vi "Teleop.vi"(10 "Match Info":T2={"Autonomous Elapsed Seconds"=0.0, "TeleOp Elapsed Seconds"=300.781, "Disabled Elapsed Seconds"=0.999, "Visited Autonomous"=FALSE, "Visited TeleOp"=TRUE, "Visited Disabled"=TRUE, "Autonomous Settings"={"Autonomous Style"=enum."Independent", "VI Refnum"=refnum}}, 11 "Call Context":T3=enum."Execute") -> ()   [LabVIEW 2016]
doc: "This VI is called for each TeleOp packet received from the DS where the robot is not disabled. It is often used to read from the joysticks and update I/O or to update setpoints for timed control loops. It should complete and return within 20 milliseconds or it may miss DS packets."
uses:
  <vilib>/Rock Robotics/WPI/DriverStation/WPI_DriverStationDerivedRobotMode.ctl
  <vilib>/Rock Robotics/WPI/DriverStation/WPI_DriverStationMatch Info.ctl
  <vilib>/Rock Robotics/WPI/Solenoid/WPI_SolenoidValue.ctl
  <vilib>/Rock Robotics/WPI/Utilities/WPI_GetSetVariantRefNum.vi
  <vilib>/Rock Robotics/Network Tables/NT Write Boolean Array.vi
  <vilib>/Rock Robotics/Network Tables/NT Write Numeric Array.vi
  <vilib>/Rock Robotics/Network Tables/NT Read Boolean.vi
  <vilib>/Rock Robotics/Network Tables/NT Read Number.vi
  <vilib>/Rock Robotics/Network Tables/NT Read String.vi
  <vilib>/Rock Robotics/WPI/Solenoid/WPI_SolenoidSetEnum.vi
  <vilib>/addons/control/pid/pid.llb/PID (DBL).vi
  <vilib>/addons/control/pid/NI_PID_pid.lvlib
panel:
  in  "PID gains":T1={"proportional gain (Kc)"=2.0, "integral time (Ti, min)"=0.02, "derivative time (Td, min)"=0.0}
  out "Output":dbl(graph)=-6.138070230177018
  out "Process Variable":dbl(graph)=160.15643445714286
  out "Setpoint":dbl(graph)=162.0
  in  "setpoint":dbl(slide)=162.0 scale=0.0..270.0
  in  "Solenoid Timer":dbl=1.0 caption="Time Target (s)"
  out "Solenoid Voltage":dbl=24.5625
  out "Input Voltage":dbl=11.45
  out "Power":dbl
  out "current (A)":dbl
  out "Degrees":dbl=160.15643445714286
  out "Voltage":dbl=2.808837603
  out "Sample Slider 0":dbl(slide) scale=0.0..5.0
  out "Sample Boolean 1":bool
  out "Sample Boolean 0":bool
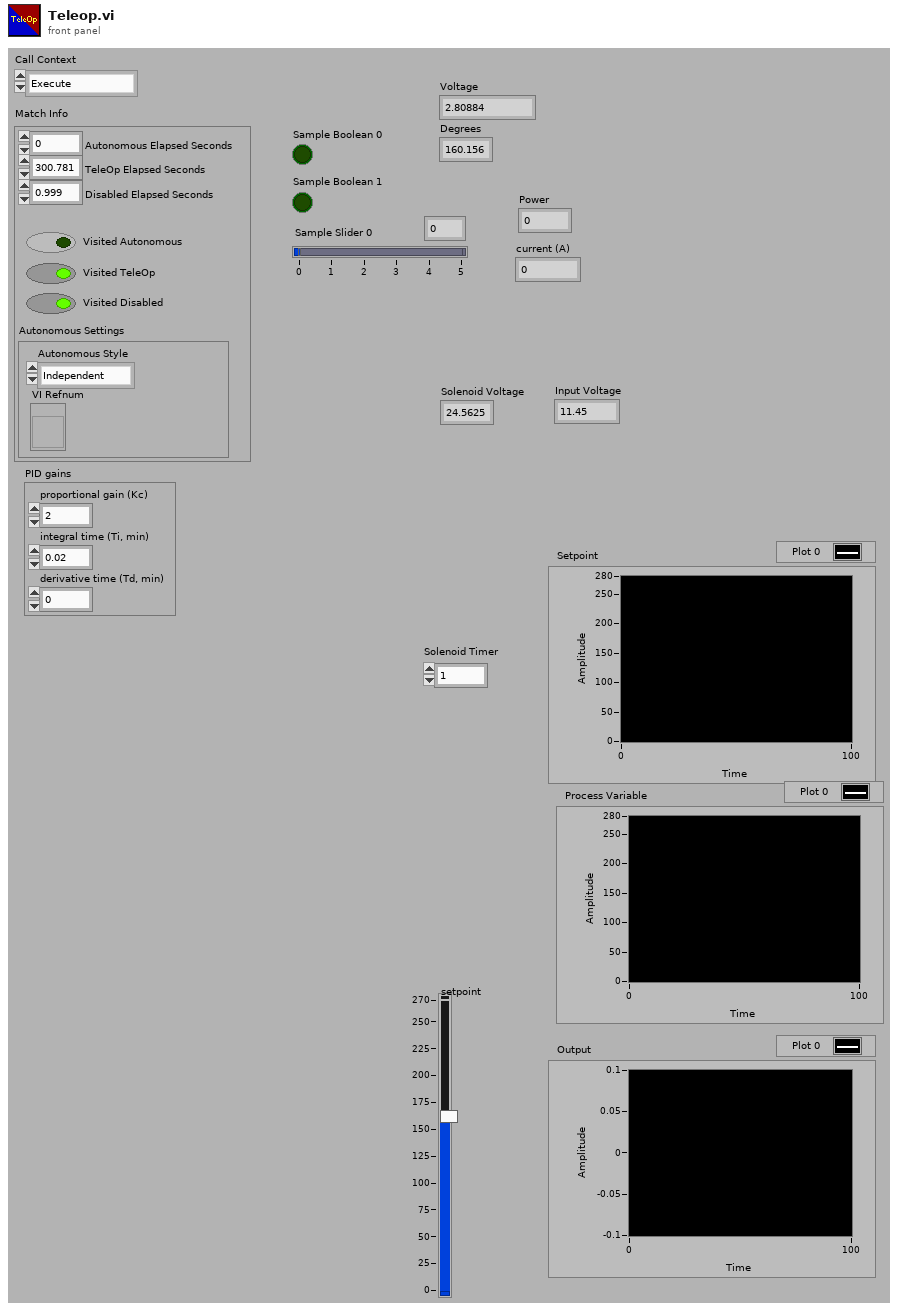
[diagram p1: front panel]
types:
  T1 = cluster{"proportional gain (Kc)":dbl, "integral time (Ti, min)":dbl, "derivative time (Td, min)":dbl}
  T2 = typedef "WPI_DriverStationMatch Info.ctl" = cluster{"Autonomous Elapsed Seconds":dbl, "TeleOp Elapsed Seconds":dbl, "Disabled Elapsed Seconds":dbl, "Visited Autonomous":bool, "Visited TeleOp":bool, "Visited Disabled":bool, "Autonomous Settings":cluster{"Autonomous Style":enum16{"Iterative", "Independent"}, "VI Refnum":refnum<vi>}}
  T3 = typedef "WPI_DriverStationDerivedRobotMode.ctl" = enum16{"Init", "Execute", "Stop"}
  T4 = typedef "WPI_SolenoidValue.ctl" = enum16{"Off", "On", "Forward", "Reverse"}
  T5 = typedef "WPI_RobotDriveDevRef.ctl" = cluster{"DevStatus":errorcluster, "Motors[]":T6[], "Square Inputs":bool, "Max Output":dbl}
  T6 = typedef "WPI_MotorControlDeviceRef.ctl" = cluster{"DeviceStatus":errorcluster, "Type":T7, "PWM":cluster{"PWM Channel":T8, "DeadBand":T9}, "CAN":cluster{"Device Number":u8, "SetOutput VI Ref":variant, "GetOutput VI Ref":variant, "Enable VI Ref":variant, "Disable VI Ref":variant, "Data":variant}, "Invert":bool}
  T7 = typedef "WPI_MotorControlType.ctl" = enum16{"PWM", "CAN"}
  T8 = typedef "FPGA_DIOPWMChannel.ctl" = enum8{"PWM 0", "PWM 1", "PWM 2", "PWM 3", "PWM 4", "PWM 5", "PWM 6", "PWM 7", "PWM 8", "PWM 9", "PWM MXP 0", "PWM MXP 1", "PWM MXP 2", "PWM MXP 3", "PWM MXP 4", "PWM MXP 5", "PWM MXP 6", "PWM MXP 7", "PWM MXP 8", "PWM MXP 9", "Invalid"}
  T9 = typedef "WPI_PWMDeadband.ctl" = cluster{"Name":string, "maxPositivePwm":i32, "minPositivePwm":i32, "centerPwm":i32, "maxNegativePwm":i32, "minNegativePwm":i32, "angularRange":u16}
  T10 = typedef "WPI_JoystickDevRef.ctl" = cluster{"Device":T11}
  T11 = typedef "WPI_JoystickDeviceEnum.ctl" = enum16{"USB 0", "USB 1", "USB 2", "USB 3", "USB 4", "USB 5"}
  T12 = typedef "WPI_AnalogChannelDevRef.ctl" = cluster{"DevStatus":errorcluster, "Analog Channel":T13}
  T13 = typedef "FPGA_AIChannel.ctl" = enum8{"AI 0", "AI 1", "AI 2", "AI 3", "AI MXP 0", "AI MXP 1", "AI MXP 2", "AI MXP 3", "Invalid"}
  T14 = typedef "WPI_SolenoidDevRef.ctl" = cluster{"DevStatus":errorcluster, "Pneumatics Control Module":u8, "Forward Solenoid Channel":T15, "Reverse Solenoid Channel":T15}
  T15 = typedef "WPI_SolenoidChannel.ctl" = enum8{"Solenoid 0", "Solenoid 1", "Solenoid 2", "Solenoid 3", "Solenoid 4", "Solenoid 5", "Solenoid 6", "Solenoid 7", "Invalid"}
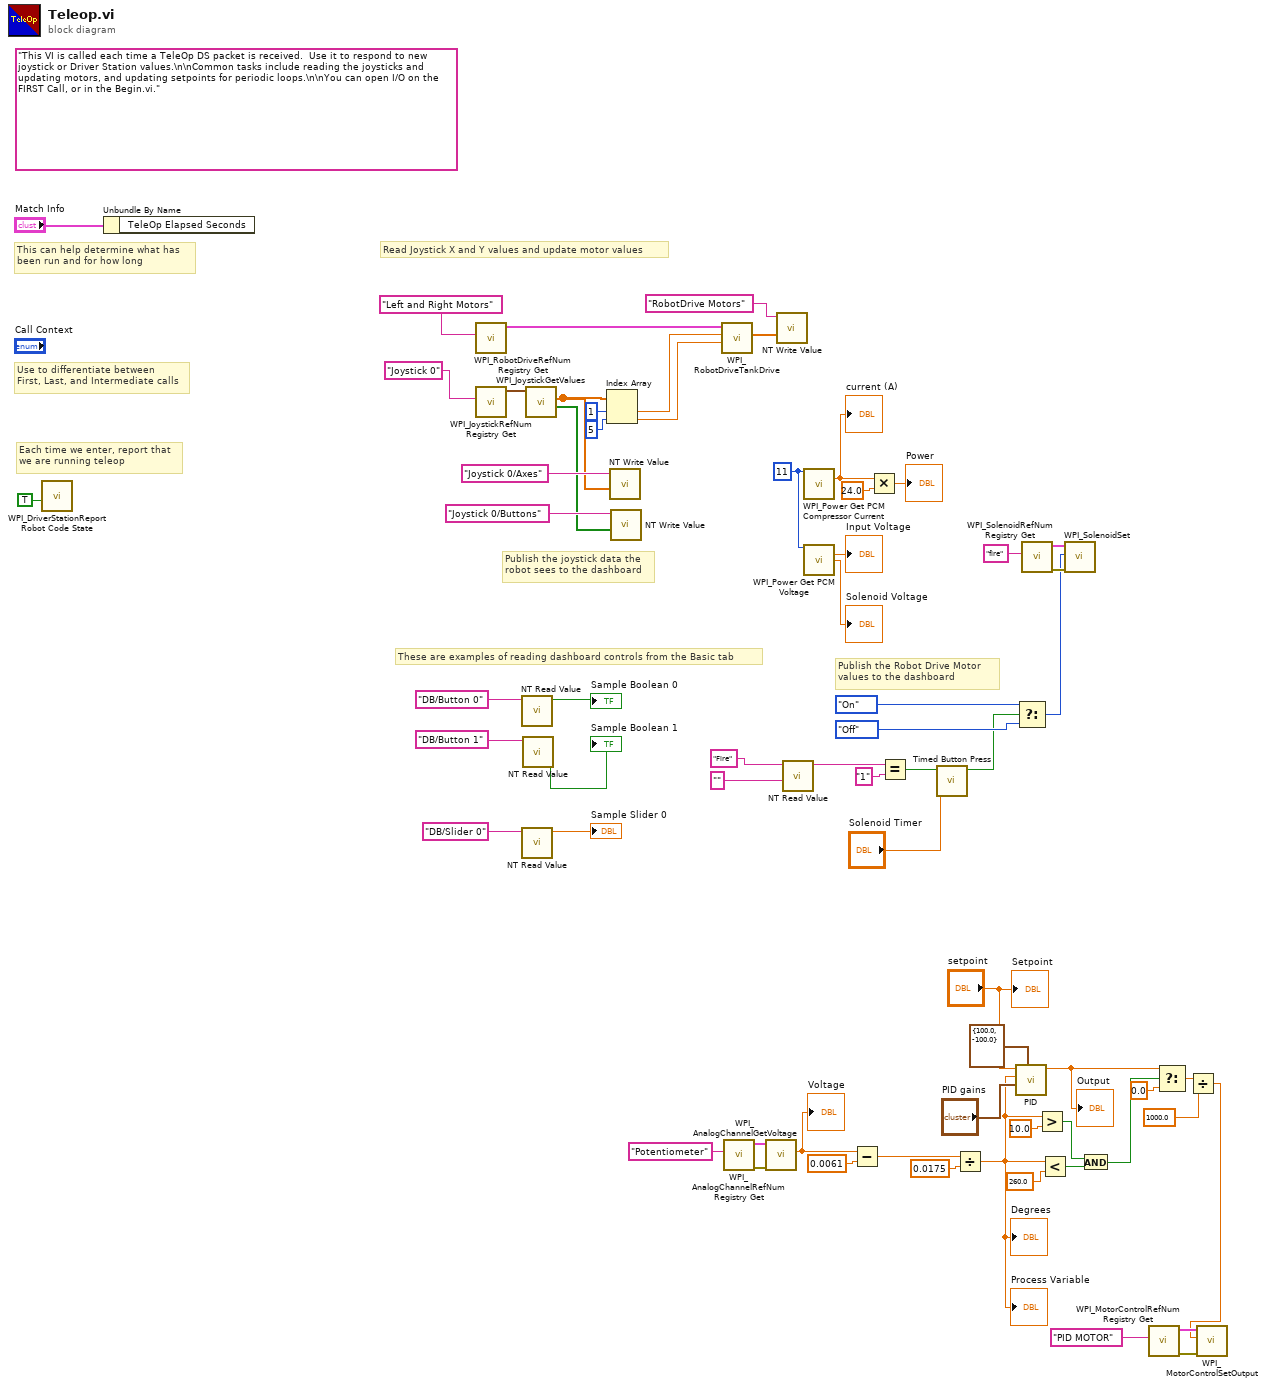
[diagram p0: block diagram]
diagram:
  w25 = u8 11 ("Pneumatics Control Module (0)")
  (unwired) "This VI is called each time a TeleOp DS packet is received.  Use it to respond to new joystick or Driver Station values.\n\nCommon tasks include reading the joysticks and updating motors, and updating setpoints for periodic loops.\n\nYou can open I/O on the FIRST Call, or in the Begin.vi."
  # "These are examples of reading dashboard controls from the Basic tab"
  # "Publish the Robot Drive Motor\nvalues to the dashboard"
  # "Publish the joystick data the\nrobot sees to the dashboard"
  # "Each time we enter, report that\nwe are running teleop"
  # "Use to differentiate between\nFirst, Last, and Intermediate calls"
  # "This can help determine what has\nbeen run and for how long"
  # "Read Joystick X and Y values and update motor values"
  n1 = call <vilib>:"WPI_DriverStationReport Robot Code State.vi"("TeleOp"=TRUE ("Autonomous")) -> ()  [unwired: 10 in, 1 out]
  n2 = Unbundle By Name("Match Info") -> ()  [unwired: 1 out]
  n3 = call <vilib>:"WPI_RobotDriveRefNum Registry Get.vi"("refnum name"="Left and Right Motors") -> ("RobotDriveDevRef"=w63:T5)  [unwired: 1 in, 9 out]
  n4 = call <vilib>:"WPI_JoystickRefNum Registry Get.vi"("refnum name"="Joystick 0") -> ("JoystickDevRef"=w60:T10)  [unwired: 1 in, 9 out]
  n5 = call-poly <vilib>:"NT Read Value.vi"("Name"="DB/Button 0" ("refnum name")) -> ("Boolean"=→"Sample Boolean 0":bool)  [unwired: 9 in, 1 out]
  n6 = call-poly <vilib>:"NT Read Value.vi"("Name"="DB/Slider 0" ("refnum name")) -> ("Numeric"=→"Sample Slider 0":dbl)  [unwired: 9 in, 1 out]
  n7 = call-poly <vilib>:"NT Read Value.vi"("Name"="DB/Button 1" ("refnum name")) -> ("Boolean"=→"Sample Boolean 1":bool)  [unwired: 9 in, 1 out]
  n8 = call <vilib>:"WPI_JoystickGetValues.vi"("JoystickDevRef"=w60) -> ("Buttons"=w32:bool[], "Axes"=w55:dbl[])  [unwired: 6 in, 3 out]
  n9 = Index Array(array=w55, index #1=1 ("index"), index #2=5 ("index")) -> (element #1=w62:dbl, element #2=w58:dbl)
  n10 = call-poly <vilib>:"NT Write Value.vi"("Numeric Array"=w55, "Name"="Joystick 0/Axes") -> ()  [unwired: 9 in, 1 out]
  n11 = call-poly <vilib>:"NT Write Value.vi"("Boolean Array"=w32, "Name"="Joystick 0/Buttons") -> ()  [unwired: 9 in, 1 out]
  n12 = call <vilib>:"WPI_RobotDriveTankDrive.vi"("Right axis value"=w58, "Left axis value"=w62, "RobotDriveDevRef"=w63) -> ("Motor Values"=w48:dbl[])  [unwired: 6 in, 2 out]
  n13 = call <vilib>:"WPI_AnalogChannelRefNum Registry Get.vi"("refnum name"="Potentiometer") -> ("error out"=w42:errorcluster, "AIDeviceRef"=w41:T12)  [unwired: 9 in]
  n14 = call <vilib>:"WPI_AnalogChannelGetVoltage.vi"("error in (no error)"=w42, "AIDeviceRef"=w41) -> ("Voltage"=w39:dbl)  [unwired: 7 in, 2 out]
  "Voltage" <- w39
  n15 = call-poly <vilib>:"NT Write Value.vi"("Numeric Array"=w48, "Name"="RobotDrive Motors") -> ()  [unwired: 9 in, 1 out]
  n16 = call-poly <vilib>:"NT Read Value.vi"("Default Value"="", "Name"="Fire") -> ("String"=w22:string)  [unwired: 8 in, 1 out]
  n17 = call <vilib>:"WPI_Power Get PCM Compressor Current.vi"("Pneumatics Control Module (0)"=w25) -> ("current (A)"=w28:dbl)  [unwired: 13 in, 1 out]
  "current (A)" <- w28
  n18 = call <vilib>:"WPI_Power Get PCM Voltage.vi"("Pneumatics Control Module (0)"=w25) -> ("Input Voltage"=→"Input Voltage":dbl, "Solenoid Voltage"=→"Solenoid Voltage":dbl)  [unwired: 12 in, 1 out]
  n19 = Subtract(x=w39, y=0.0061) -> (x-y=w37:dbl)
  n20 = Multiply(x=w28, y=24.0) -> (x*y=→"Power":dbl)
  n21 = Equal?(x=w22, y="1") -> (x = y?=w19:bool)
  n22 = call "Timed Button Press.vi"("Time Target (s)"="Solenoid Timer", "Boolean 2"=w19) -> ("Boolean"=w20:bool)  [unwired: 9 in]
  n23 = Divide(x=w37, y=0.0175) -> (x/y=w5:dbl)
  "Degrees" <- w5
  "Process Variable" <- w5
  n24 = call-poly <vilib>:"PID.vi"("output range"=cluster{"output high":dbl, "output low":dbl} {"output high"=100.0, "output low"=-100.0}, "PID gains"="PID gains", "process variable"=w5, "setpoint"="setpoint") -> ("output"=w10:dbl)  [unwired: 6 in, 1 out]
  "Output" <- w10
  n25 = Select(t=WPI_SolenoidValue."On" ("Value"), s=w20, f=WPI_SolenoidValue."Off" ("Value")) -> (s? t:f=w30:T4)
  n26 = call <vilib>:"WPI_SolenoidRefNum Registry Get.vi"("refnum name"="fire") -> ("error out"=w33:errorcluster, "SolenoidDevRef"=w34:T14)  [unwired: 9 in]
  n27 = Greater?(x=w5, y=10.0) -> (0:w9:bool)
  n28 = Less?(x=w5, y=260.0) -> (x < y?=w8:bool)
  n29 = call-poly <vilib>:"WPI_SolenoidSet.vi"("error in (no error)"=w33, "Value"=w30, "SolenoidDevRef"=w34) -> ()  [unwired: 7 in, 2 out]
  n30 = And(x=w9, y=w8) -> (x .and. y?=w11:bool)
  n31 = call <vilib>:"WPI_MotorControlRefNum Registry Get.vi"("refnum name"="PID MOTOR") -> ("error out"=w13:errorcluster, "MotorControlDevRef"=w12:T6)  [unwired: 9 in]
  n32 = Select(t=w10, s=w11, f=0.0) -> (s? t:f=w3:dbl)
  n33 = Divide(x=w3, y=1000.0) -> (x/y=w1:dbl)
  n34 = call <vilib>:"WPI_MotorControlSetOutput.vi"("error in (no error)"=w13, "Output"=w1, "MotorControlDevRef"=w12) -> ()  [unwired: 6 in, 3 out]
  "Setpoint" <- "setpoint"
